vi "test_victor_linearize.vi"() -> ()   [LabVIEW 2011]
panel:
  out "XY Graph":cluster{"X":dbl, "Y":dbl}[](graph)
  out "i":dbl
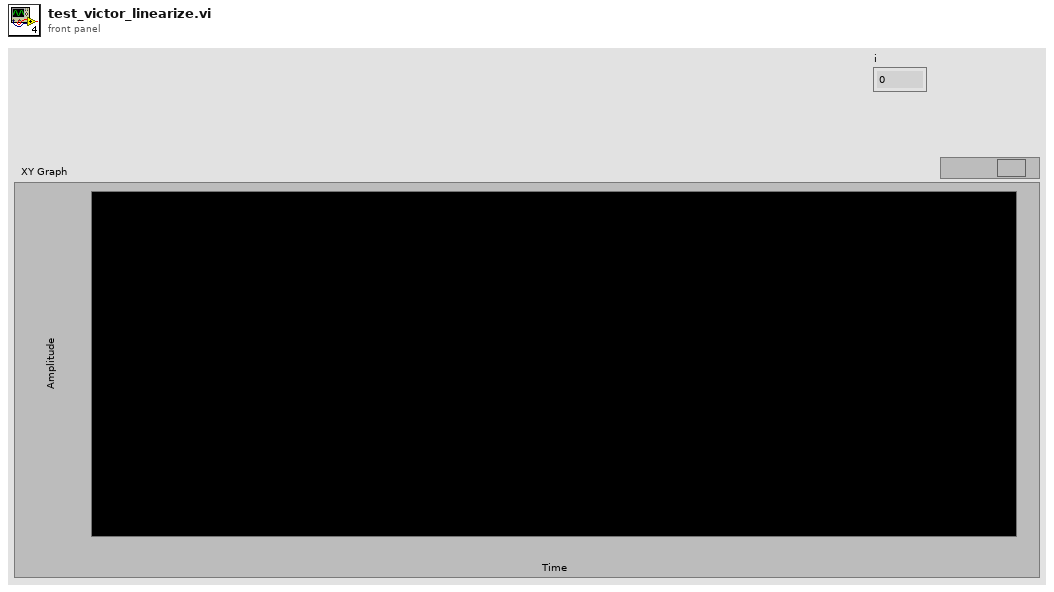
[diagram p1: front panel]
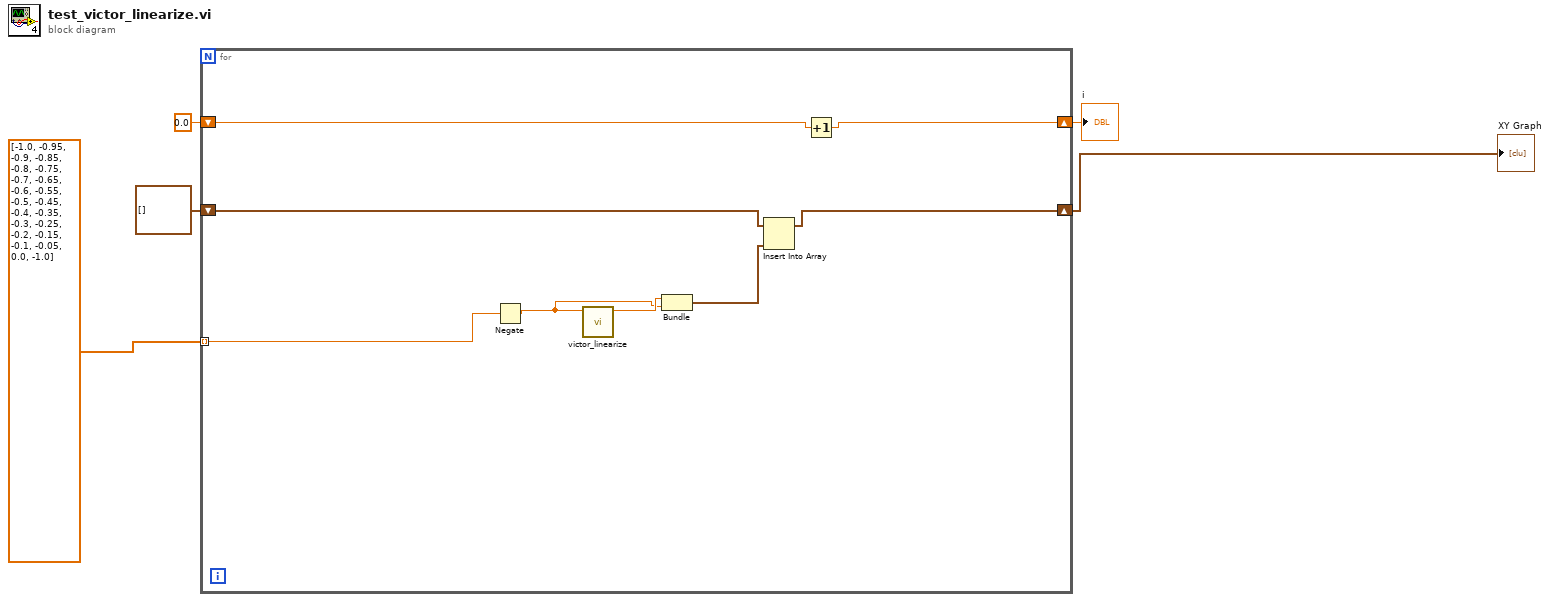
[diagram p0: block diagram]
diagram:
  n1 = for {
    tunnel: dbl[] [-1.0, -0.95, -0.9, -0.85, -0.8, -0.75, -0.7, -0.65, -0.6, -0.55, -0.5, -0.45, -0.4, -0.35, -0.3, -0.25, -0.2, -0.15, -0.1, -0.05, 0.0, -1.0] -> [w8] mode=indexing
    shift-right: [w11] -> w1
    shift-left: cluster{dbl, "Output":dbl}[] [] -> [w12]
    shift-right: [w10] -> w3
    shift-left: 0.0 -> [w9]
    n2 = Negate(x=w8) -> (-x=w6:dbl)
    n3 = call "victor_linearize.vi"("Input"=w6) -> ("Output"=w7:dbl)  [unwired: 10 in]
    n4 = Bundle("Output"=w7, w6) -> (w13:cluster{"Output":dbl, dbl})  [unwired: 1 in]
    n5 = Insert Into Array(array=w12, new element=w13) -> (w11:cluster{dbl, "Output":dbl}[])  [unwired: 1 in]
    n6 = Increment(x=w9) -> (x+1=w10:dbl)
  }
  "i" <- w3
  "XY Graph" <- w1
